vi "Control Pump Power (acc and temp).vi"(0 "CAN Session In":T1, 1 "Pumps power in":dbl(slide) scale=0.0..100.0 scale format="%#_g%%", 2 "\"Pedals\" Status":T2 {"Acceleration pedal" scale=0.0..100.0 scale format="%#_6f%%"; "Break pedal" scale=0.0..100.0 scale format="%#_6f%%"}, 3 "Left Motor Status":T3, 4 "Right Motor Status":T3, 5 "error in":errorcluster, 6 "Simulate Pumps":bool, 8 "timeout":i32=1000) -> (14 "CAN Session Out":T1, 15 "Pumps power out":dbl(slide) scale=0.0..100.0 scale format="%#_g%%", 19 "error out":errorcluster)   [LabVIEW 2016]
uses:
  RT/Pedals Status.ctl
  Program Files (x86)/National Instruments/LabVIEW 2016/examples/robotics/EPOS2 CANOpen Driver/Low Level VIs/Typedefs/CAN Refnum.ctl
  Program Files (x86)/National Instruments/LabVIEW 2016/examples/robotics/EPOS2 CANOpen Driver/Low Level VIs/Typedefs/CAN Session Pointer.ctl
  Program Files (x86)/National Instruments/LabVIEW 2016/examples/robotics/EPOS2 CANOpen Driver/Low Level VIs/Typedefs/CAN Communication References.ctl
  Program Files (x86)/National Instruments/LabVIEW 2016/examples/robotics/EPOS2 CANOpen Driver/Low Level VIs/Typedefs/kill process notifier array.ctl
  Program Files (x86)/National Instruments/LabVIEW 2016/examples/robotics/EPOS2 CANOpen Driver/Low Level VIs/Typedefs/Write Queue.ctl
  Program Files (x86)/National Instruments/LabVIEW 2016/examples/robotics/EPOS2 CANOpen Driver/Low Level VIs/Typedefs/FPGA CAN Frame Cluster.ctl
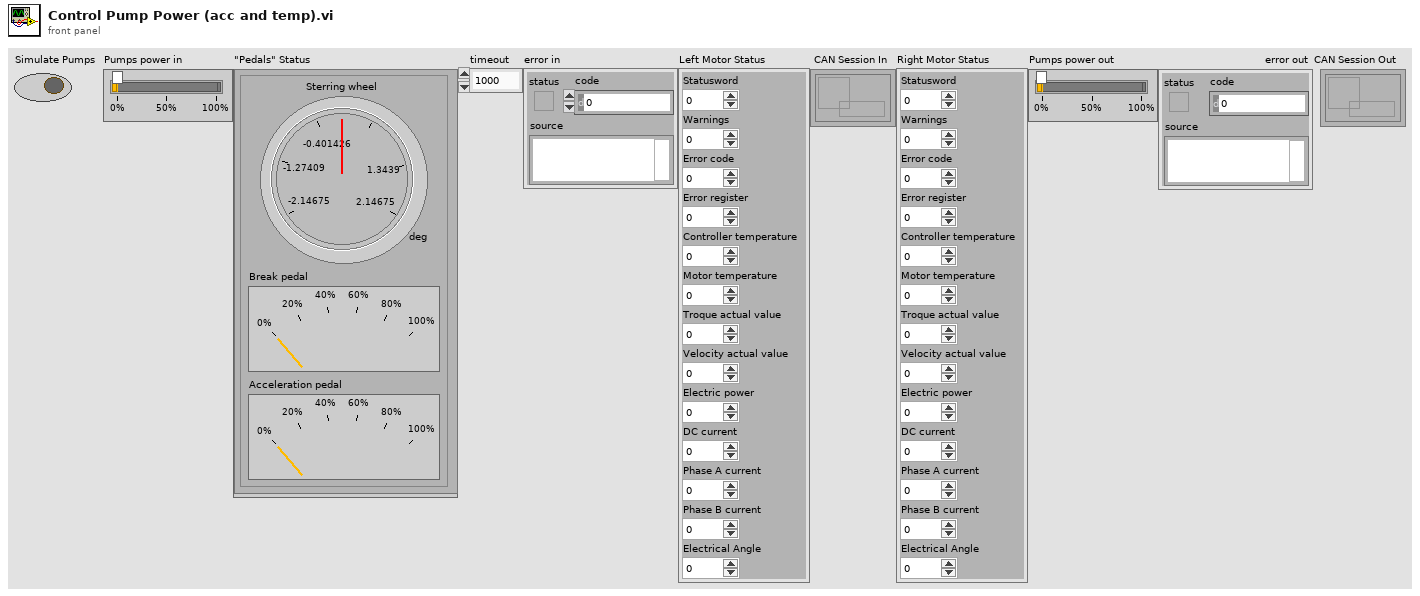
[diagram p1: front panel]
types:
  T1 = typedef "CAN Refnum.ctl" = refnum<k1>
  T2 = typedef "Pedals Status.ctl" = cluster{"Acceleration pedal":dbl, "Break pedal":dbl, "Sterring wheel":dbl[unit]}
  T3 = cluster{"Statusword":u16, "Warnings":u16, "Error code":u16, "Error register":u8, "Controller temperature":u8, "Motor temperature":u8, "Troque actual value":i16, "Velocity actual value":i32, "Electric power":u32, "DC current":u32, "Phase A current":u16, "Phase B current":u16, "Electrical Angle":u16}
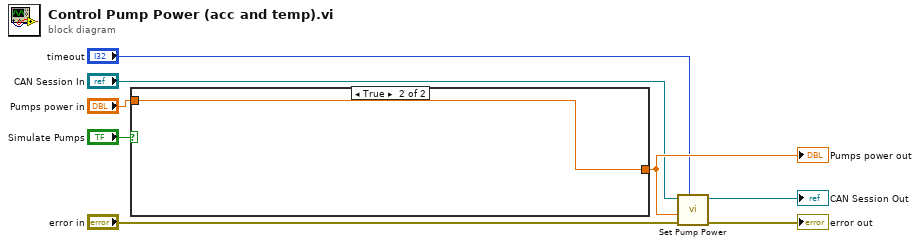
[diagram p0: block diagram]
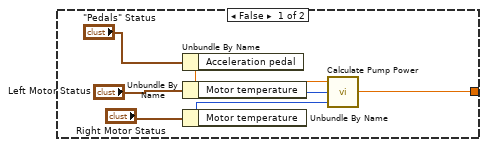
[diagram p2: hidden frame]
diagram:
  n1 = case shown="True" "Simulate Pumps" {
    tunnel: [w12 w16] -> w7
    tunnel: "Pumps power in" -> [_ w16]
    frame False {
      n2 = Unbundle By Name("\"Pedals\" Status") -> ("Acceleration pedal"=w13:dbl)
      n3 = Unbundle By Name("Left Motor Status") -> ("Motor temperature"=w14:u8)
      n4 = Unbundle By Name("Right Motor Status") -> ("Motor temperature"=w15:u8)
      n5 = call "Calculate Pump Power.vi"("Motor temperature 2"=w15, "Motor temperature"=w14, "Acceleration pedal"=w13) -> ("Pumps power"=w12:dbl)
    }
    frame True {
    }
  }
  "Pumps power out" <- w7
  n6 = call "Set Pump Power.vi"("timeout"="timeout", "error in"="error in", "Power %"=w7, "CAN Session In"="CAN Session In") -> ("error out"=→"error out":errorcluster, "CAN Session Out"=→"CAN Session Out":T1)  [unwired: 6 in]
